vi "3.4-4.7.4-How Server.vi"() -> ()   [LabVIEW 2010]
doc: "UDP Mutlicast Addressing Scheme:\n\n3.7 - Multicast Address: 224.0.3.7\n3.1-4.7.1 Port: 31471\n3.2-4.7.2 Port: 32472\n3.3-4.7.3 Port: 33473\n3.4-4.7.4 Port: 34474\n\n5.7 - Multicast Address: 224.0.5.7\n5.1-4.7.1 Port: 51471\n5.2-4.7.2 Port: 52472\n5.3-4.7.3 Port: 53473\n5.4-4.7.4 Port: 54474\n\n5.1-6.7.1 Port: 51671\n5.2-6.7.2 Port: 52672\n5.3-6.7.3 Port: 53673\n5.4-6.7.4 Port: 54674\n\n7.7 - Multicast Address: 224.0.7.7\n7.1-6.7.1 Port: 61671\n7.2-6.7.2 Port: 62672\n7.3-6.7.3 Port: 63673\n7.4-6.7.4 Port: 64674"
uses:
  4-High Neurons/4.0-Timing Badass.ctl
  3.7-UDP/3.7-UDP Make Checksum.vi
  <vilib>/Utility/tcp.llb/UDP Multicast Write-Only Open.vi
  3.0-Global.vi
panel:
  out "Super Heart Beat":T1
  out "Error":errorcluster
  in  "stop":bool
  out "Processed":string
  in  "Debug Data":string
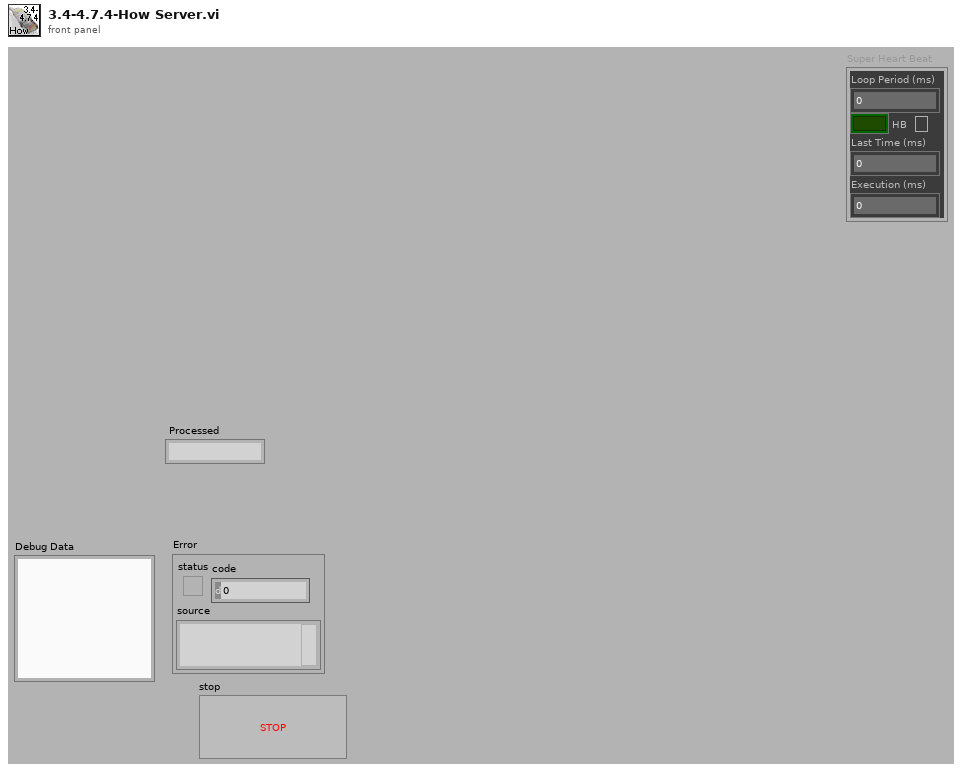
[diagram p1: front panel]
types:
  T1 = typedef "4.0-Timing Badass.ctl" = cluster{"Loop Period (ms)":u32, "HB":bool, "Last Time (ms)":u32, "Execution (ms)":u32}
  T2 = typedef "4.4-How Sensor Typedef.ctl" = cluster{"Motor Speed Integer":i32, "Drive Position Integer":i32, "Lidar Position Integer":i32, "Lidar Motor Position Integer":i32, "Steering Position Integer":i32, "Battery Voltage Fxp":dbl, "Drive Encoder Cable Check":bool, "Lidar Drive Encoder Cable Check":bool, "Steer Encoder Cable Check":bool, "Lidar Pos Encoder Cable Check":bool, "Mod Buttons & Blinky Cable Check":bool, "Lidar Data Cable Check":bool, "Drive Motor Cable Check":bool, "Vector Nav Cable Check":bool, "Lidar Drive Cable Check":bool, "Steer Drive Cable Check":bool, "Reverse?":bool, "2.1  Steering Control Voltage":dbl, "2.1 Drive Control Voltage":dbl, "2.1  Lidar Control Voltage":dbl, "2.5.7 A*B":dbl, "2.1  Steering PID Output":dbl, "2.1 Drive PID Output":dbl, "2.1  Lidar PID Output":dbl, "2.1.1 Drive Error":dbl, "2.1.1 Drive Error I":dbl, "2.1.1 Drive Error D":dbl, "2.1.2 Steering Error":dbl, "2.1.2 Steering Error I":dbl, "2.1.2 Steering Error D":dbl, "2.1.3 Lidar Error":dbl, "2.1.3 Lidar Error I":dbl, "2.1.3 Lidar Error D":dbl, "VectorNav Ack Query":bool, "VectorNav Read Byte":u8, "VectorNav Read Status":enum16{"Waiting", "Reading", "Done"}, "4.0-Midbrain State":T3}
  T3 = typedef "4.0-Midbrain State.ctl" = enum16{"Startup", "Waiting to Run", "Running-OlinOval", "Running-ChannelFollow", "Running-WallFollow", "Running-OpenTransit", "Running-Joystick Training", "Shutdown", "Restart"}
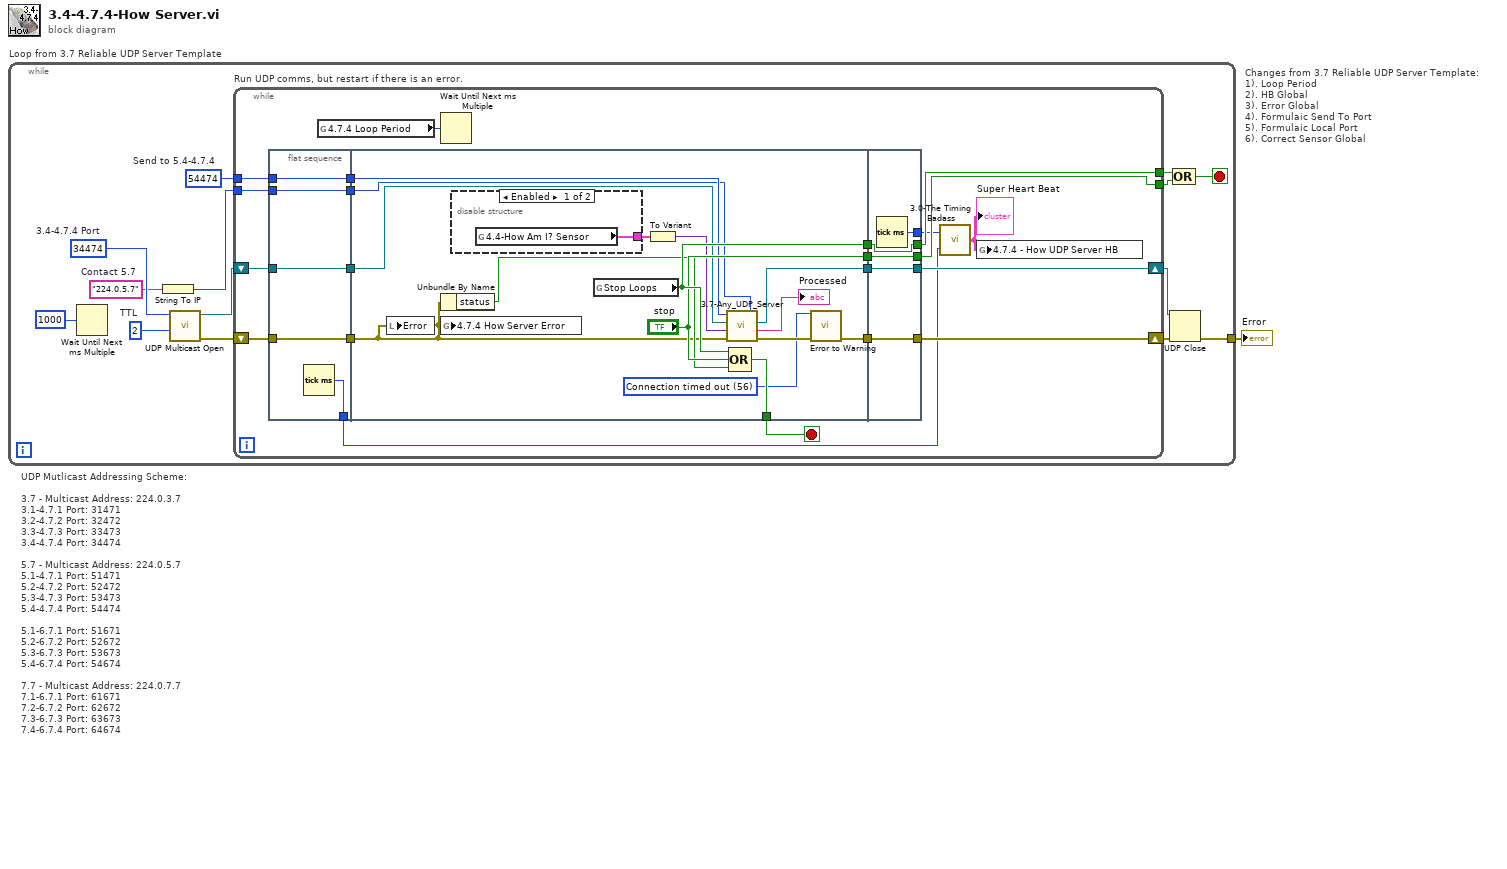
[diagram p0: block diagram]
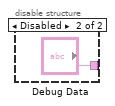
[diagram p2: hidden frame]
diagram:
  # "Changes from 3.7 Reliable UDP Server Template:\n1). Loop Period\n2). HB Global\n3). Error Global\n4). Formulaic Send To Port\n5). Formulaic Local Port\n6). Correct Sensor Global"
  # "UDP Mutlicast Addressing Scheme:\n\n3.7 - Multicast Address: 224.0.3.7\n3.1-4.7.1 Port: 31471\n3.2-4.7.2 Port: 32472\n3.3-4.7.3 Port: 33473\n3.4-4.7.4 Port: 34474\n\n5.7 - Multicast Address: 224.0.5.7\n5.1-4.7.1 Port: 51471\n5.2-4.7.2 Port: 52472\n5.3-4.7.3 Port: 53473\n5.4-4.7.4 Port: 54474\n\n5.1-6.7.1 Port: 51671\n5.2-6.7.2 Port: 52672\n5.3-6.7.3 Port: 53673\n5.4-6.7.4 Port: 54674\n\n7.7 - Multicast Address: 224.0.7.7\n7.1-6.7.1 Port: 61671\n7.2-6.7.2 Port: 62672\n7.3-6.7.3 Port: 63673\n7.4-6.7.4 Port: 64674"
  n1 = while "Loop from 3.7 Reliable UDP Server Template" {
    tunnel: [w10] -> w1
    stop <- w13 stop-if-true
    w2 = "224.0.5.7"  # Contact 5.7
    w4 = u16 54474  # Send to 5.4-4.7.4
    w7 = u16 2  # TTL
    w8 = u16 34474  # 3.4-4.7.4 Port
    n2 = Wait Until Next ms Multiple(millisecond multiple=u32 1000) -> ()  [unwired: 1 out]
    n3 = String To IP(1:w2) -> (0:w3:u32)
    n4 = call-poly <vilib>:"UDP Multicast Open.vi"("time-to-live (1)"=w7, "port"=w8) -> ("error out"=w5:errorcluster, "connection ID"=w6:refnum<k16>)  [unwired: 8 in]
    n5 = while "Run UDP comms, but restart if there is an error." {
      tunnel: [w35] -> w15
      tunnel: [w34] -> w14
      shift-right: [w31] -> w12
      shift-left: w6 -> [w32]
      shift-right: [w28] -> w11
      shift-left: w5 -> [w33]
      tunnel: w4 -> [w30]
      tunnel: w3 -> [w29]
      stop <- w36 stop-if-true
      n6 = flat-sequence {
        tunnel: w29 -> [w38]
        tunnel: w30 -> [w39]
        tunnel: w32 -> [w40]
        tunnel: w33 -> [w41]
        tunnel: [w41] -> w22
        tunnel: [w40] -> w21
        tunnel: [w39] -> w20
        tunnel: [w38] -> w19
        tunnel: [w37] -> w17
        tunnel: [w56] -> w36
        tunnel: [w55] -> w26
        tunnel: ["stop"] -> w25
        tunnel: [w47] -> w24
        tunnel: [w42] -> w23
        tunnel: w22 -> [w51]
        tunnel: w21 -> [w48]
        tunnel: w20 -> [w46]
        tunnel: w19 -> [w45]
        tunnel: [w60] -> w28
        tunnel: [w61] -> w31
        tunnel: [w62] -> w34
        tunnel: [w63] -> w35
        tunnel: w26 -> [w63]
        tunnel: w25 -> [w62]
        tunnel: w24 -> [w61]
        tunnel: w23 -> [w60]
        tunnel: [w59] -> w18
        frame #0 {
          n7 = Tick Count (ms)() -> (millisecond timer value=w37:u32)
        }
        frame #1 {
          w43 = 56 items=["No Error", "Argument Error", "Memory Full", "Out of Zone", "End of File", "File Already Open", "Generic File IO Error", "File Not Found", "File Permission Error", "Disk Full", "Duplicate Path", "Too Many Files Open", "Not Enabled", "Resource File Not Found", "Cannot Add Resource", "Resource Not Found", "Image Not Found", "Image Memory Error", "Pen Does Not Exist", "Config Bad Type", "Config Token Not Found", "Config Parse Error", "Config Memory Error", "Bad External Code Format", "Bad External Code Offset", "External Code Not Present", "Null Window", "Destroy Window Mixup", "Null Menu", "Print Aborted", "Bad Print Record", "Print Driver Error", "Windows Error During Print", "Memory Error During Print", "Print Dialog Error", "Generic Print Error", "Invalid Device Refnum", "Device Not Found", "Device Parameter Error", "Device Unit Error", "Can't Open Device", "Device Call Aborted", "Generic Error", "Cancelled By User", "Object ID Too Low", "Object ID Too High", "Object Not In Heap", "Unknown Heap", "Bad DefProc ID", "DefProc Not In Table", "Message Out Of Range", "Null Method", "Unknown Message", "Manager Call Not Supported", "Bad address", "Connection In progress", "Connection timed out", "Connection is already in progress", "Network attribute not supported", "Network error", "Address in use", "System out of memory", "Connection aborted", "Connection refused", "Connection is not connected", "Connection is already connected", "Connection closed", "Initialize error (interapplication manager)", "Bad occurrence", "Wait on unbound occurrence handler", "Occurrence queue overflow", "Bad path", "Semaphore not signaled", "Unrecognized type (interapplication manager)"] ("1st Error to Convert")
          n8 = local write "Error"(w51) -> ()
          n9 = Unbundle By Name(w51) -> ("status"=w53:bool)
          n10 = global write "3.0-Global.vi" "4.7.4 How Server Error"(w51) -> ()
          n11 = disable-structure shown="Enabled" {
            disable-tunnel: [w57 "Debug Data"] -> w50
            frame Enabled {
              n12 = global read "3.0-Global.vi" "4.4-How Am I? Sensor"() -> (w57:T2)
            }
            frame Disabled {
            }
          }
          n13 = global read "3.0-Global.vi" "Stop Loops"() -> (w55:bool)
          n14 = To Variant(anything=w50) -> (Variant=w52:variant)
          n15 = call "3.7-Any_UDP_Server.vi"("Multicast Address"=w45, "error In"=w51, "Data in"=w52, "Connection ID"=w48, "Send To Port"=w46) -> ("warning out"=w44:errorcluster, "Processed"=→"Processed":string, "Connection ID out"=w47:refnum<k16>)
          n16 = Compound Arithmetic op=OR(w55, "stop", w53) -> (w56:bool)
          n17 = call <vilib>:"Error to Warning.vi"("1st Error to Convert"=w43, "error in"=w44) -> ("warning out"=w42:errorcluster)  [unwired: 13 in]
        }
        frame #2 {
          n18 = Tick Count (ms)() -> (millisecond timer value=w59:u32)
        }
      }
      n19 = global read "3.0-Global.vi" "4.7.4 Loop Period"() -> (w27:u32)
      n20 = Wait Until Next ms Multiple(millisecond multiple=w27) -> ()  [unwired: 1 out]
      n21 = call "3.0-The Timing Badass.vi"("Start"=w17, "End"=w18) -> ("Super Heart Beat"=w16:T1)
      "Super Heart Beat" <- w16
      n22 = global write "3.0-Global.vi" "4.7.4 - How UDP Server HB"(w16) -> ()
    }
    n23 = UDP Close(connection ID=w12, 8:w11) -> (error out=w10:errorcluster)  [unwired: 1 out]
    n24 = Compound Arithmetic op=OR(w15, w14) -> (w13:bool)
  }
  "Error" <- w1
